vi "MCCETC_Status.vi"() -> (0 "n_ng":u8, 1 "values3":T1, 2 "values2":T2, 3 "values1":T3)   [LabVIEW 2019]
uses:
  MCCETC_Global.vi
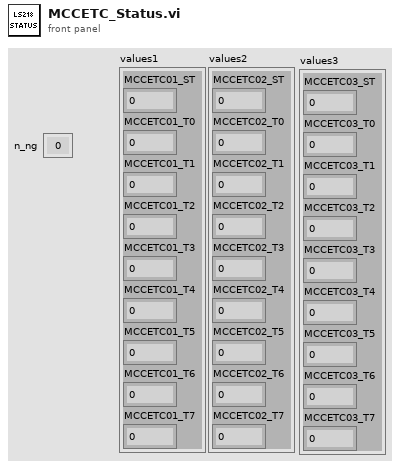
[diagram p1: front panel]
types:
  T1 = cluster{"MCCETC03_ST":u32, "MCCETC03_T0":dbl, "MCCETC03_T1":dbl, "MCCETC03_T2":dbl, "MCCETC03_T3":dbl, "MCCETC03_T4":dbl, "MCCETC03_T5":dbl, "MCCETC03_T6":dbl, "MCCETC03_T7":dbl}
  T2 = cluster{"MCCETC02_ST":u32, "MCCETC02_T0":dbl, "MCCETC02_T1":dbl, "MCCETC02_T2":dbl, "MCCETC02_T3":dbl, "MCCETC02_T4":dbl, "MCCETC02_T5":dbl, "MCCETC02_T6":dbl, "MCCETC02_T7":dbl}
  T3 = cluster{"MCCETC01_ST":u32, "MCCETC01_T0":dbl, "MCCETC01_T1":dbl, "MCCETC01_T2":dbl, "MCCETC01_T3":dbl, "MCCETC01_T4":dbl, "MCCETC01_T5":dbl, "MCCETC01_T6":dbl, "MCCETC01_T7":dbl}
  T4 = enum32{"Bad", "Idle", "Run top level", "Running"}
  T5 = cluster{"MKS670_1000_ST":u32, "MCCETC03_T0":dbl, "MCCETC03_T1":dbl, "MCCETC03_T2":dbl, "MCCETC03_T3":dbl, "MCCETC03_T4":dbl, "MCCETC03_T5":dbl, "MCCETC03_T6":dbl, "MCCETC03_T7":dbl}
  T6 = cluster{"MKS670_1000_ST":u32, "MCCETC02_T0":dbl, "MCCETC02_T1":dbl, "MCCETC02_T2":dbl, "MCCETC02_T3":dbl, "MCCETC02_T4":dbl, "MCCETC02_T5":dbl, "MCCETC02_T6":dbl, "MCCETC02_T7":dbl}
  T7 = cluster{"MKS670_1000_ST":u32, "MCCETC01_T0":dbl, "MCCETC01_T1":dbl, "MCCETC01_T2":dbl, "MCCETC01_T3":dbl, "MCCETC01_T4":dbl, "MCCETC01_T5":dbl, "MCCETC01_T6":dbl, "MCCETC01_T7":dbl}
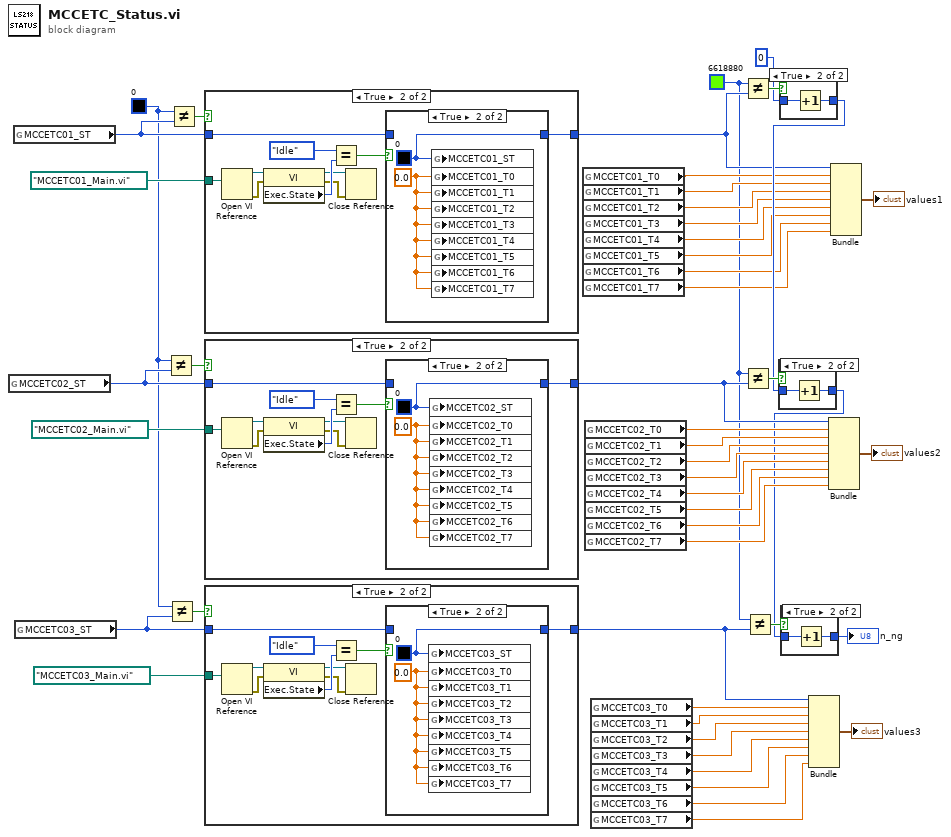
[diagram p0: block diagram]
diagram:
  w16 = u32 6618880 ("MKS670_1000_ST 2")
  w17 = u32 0 ("MKS670_1000_ST 2")
  n1 = global read "MCCETC_Global.vi" "MCCETC02_ST"() -> (w37:u32)
  n2 = global read "MCCETC_Global.vi" "MCCETC01_ST"() -> (w38:u32)
  n3 = global read "MCCETC_Global.vi" "MCCETC03_ST"() -> (w18:u32)
  n4 = Not Equal?(x=w17, y=w37) -> (x != y?=w46:bool)
  n5 = Not Equal?(x=w17, y=w18) -> (x != y?=w19:bool)
  n6 = Not Equal?(x=w17, y=w38) -> (x != y?=w48:bool)
  n7 = case shown="True" w48 {
    tunnel: w38 -> [w49 w51]
    tunnel: [w49 w50] -> w40
    tunnel: path "MCCETC01_Main.vi" ("vi path") -> [_ w52]
    frame False {
    }
    frame True {
      n8 = Open VI Reference(vi path=w52) -> (vi reference=w59:refnum<vi>, error out=w58:errorcluster)  [unwired: 5 in]
      n9 = property class="VI"(reference=w59, error in=w58) -> (reference out=w54:refnum<vi>, error out=w53:errorcluster, "Exec.State"=w56:T4)
      n10 = Equal?(x=T4."Idle" ("Execution:State"), y=w56) -> (x = y?=w57:bool)
      n11 = Close Reference(reference=w54, error in (no error)=w53) -> ()  [unwired: 1 out]
      n12 = case shown="True" w57 {
        tunnel: w51 -> [w60 _]
        tunnel: [w60 w62] -> w50
        frame False {
        }
        frame True {
          w61 = 0.0 ("MKS670_1000_P")
          w62 = u32 0 ("MKS670_1000_ST")
          n13 = global write "MCCETC_Global.vi" "MCCETC01_ST"(w62) -> ()
          n14 = global write "MCCETC_Global.vi" "MCCETC01_T0"(w61) -> ()
          n15 = global write "MCCETC_Global.vi" "MCCETC01_T1"(w61) -> ()
          n16 = global write "MCCETC_Global.vi" "MCCETC01_T2"(w61) -> ()
          n17 = global write "MCCETC_Global.vi" "MCCETC01_T3"(w61) -> ()
          n18 = global write "MCCETC_Global.vi" "MCCETC01_T4"(w61) -> ()
          n19 = global write "MCCETC_Global.vi" "MCCETC01_T5"(w61) -> ()
          n20 = global write "MCCETC_Global.vi" "MCCETC01_T6"(w61) -> ()
          n21 = global write "MCCETC_Global.vi" "MCCETC01_T7"(w61) -> ()
        }
      }
    }
  }
  n22 = case shown="True" w46 {
    tunnel: w37 -> [w63 w65]
    tunnel: [w63 w64] -> w39
    tunnel: path "MCCETC02_Main.vi" ("vi path") -> [_ w66]
    frame False {
    }
    frame True {
      n23 = Open VI Reference(vi path=w66) -> (vi reference=w73:refnum<vi>, error out=w72:errorcluster)  [unwired: 5 in]
      n24 = property class="VI"(reference=w73, error in=w72) -> (reference out=w68:refnum<vi>, error out=w67:errorcluster, "Exec.State"=w70:T4)
      n25 = Equal?(x=T4."Idle" ("Execution:State"), y=w70) -> (x = y?=w71:bool)
      n26 = Close Reference(reference=w68, error in (no error)=w67) -> ()  [unwired: 1 out]
      n27 = case shown="True" w71 {
        tunnel: w65 -> [w74 _]
        tunnel: [w74 w76] -> w64
        frame False {
        }
        frame True {
          w75 = 0.0 ("MKS670_1000_P")
          w76 = u32 0 ("MKS670_1000_ST")
          n28 = global write "MCCETC_Global.vi" "MCCETC02_ST"(w76) -> ()
          n29 = global write "MCCETC_Global.vi" "MCCETC02_T0"(w75) -> ()
          n30 = global write "MCCETC_Global.vi" "MCCETC02_T1"(w75) -> ()
          n31 = global write "MCCETC_Global.vi" "MCCETC02_T2"(w75) -> ()
          n32 = global write "MCCETC_Global.vi" "MCCETC02_T3"(w75) -> ()
          n33 = global write "MCCETC_Global.vi" "MCCETC02_T4"(w75) -> ()
          n34 = global write "MCCETC_Global.vi" "MCCETC02_T5"(w75) -> ()
          n35 = global write "MCCETC_Global.vi" "MCCETC02_T6"(w75) -> ()
          n36 = global write "MCCETC_Global.vi" "MCCETC02_T7"(w75) -> ()
        }
      }
    }
  }
  n37 = case shown="True" w19 {
    tunnel: w18 -> [w77 w79]
    tunnel: [w77 w78] -> w12
    tunnel: path "MCCETC03_Main.vi" ("vi path") -> [_ w80]
    frame False {
    }
    frame True {
      n38 = Open VI Reference(vi path=w80) -> (vi reference=w87:refnum<vi>, error out=w86:errorcluster)  [unwired: 5 in]
      n39 = property class="VI"(reference=w87, error in=w86) -> (reference out=w82:refnum<vi>, error out=w81:errorcluster, "Exec.State"=w84:T4)
      n40 = Equal?(x=T4."Idle" ("Execution:State"), y=w84) -> (x = y?=w85:bool)
      n41 = Close Reference(reference=w82, error in (no error)=w81) -> ()  [unwired: 1 out]
      n42 = case shown="True" w85 {
        tunnel: w79 -> [w88 _]
        tunnel: [w88 w90] -> w78
        frame False {
        }
        frame True {
          w89 = 0.0 ("MKS670_1000_P")
          w90 = u32 0 ("MKS670_1000_ST")
          n43 = global write "MCCETC_Global.vi" "MCCETC03_ST"(w90) -> ()
          n44 = global write "MCCETC_Global.vi" "MCCETC03_T0"(w89) -> ()
          n45 = global write "MCCETC_Global.vi" "MCCETC03_T1"(w89) -> ()
          n46 = global write "MCCETC_Global.vi" "MCCETC03_T2"(w89) -> ()
          n47 = global write "MCCETC_Global.vi" "MCCETC03_T3"(w89) -> ()
          n48 = global write "MCCETC_Global.vi" "MCCETC03_T4"(w89) -> ()
          n49 = global write "MCCETC_Global.vi" "MCCETC03_T5"(w89) -> ()
          n50 = global write "MCCETC_Global.vi" "MCCETC03_T6"(w89) -> ()
          n51 = global write "MCCETC_Global.vi" "MCCETC03_T7"(w89) -> ()
        }
      }
    }
  }
  n52 = global read "MCCETC_Global.vi" "MCCETC01_T0"() -> (w36:dbl)
  n53 = global read "MCCETC_Global.vi" "MCCETC01_T1"() -> (w35:dbl)
  n54 = global read "MCCETC_Global.vi" "MCCETC01_T2"() -> (w34:dbl)
  n55 = global read "MCCETC_Global.vi" "MCCETC01_T3"() -> (w33:dbl)
  n56 = global read "MCCETC_Global.vi" "MCCETC01_T4"() -> (w32:dbl)
  n57 = global read "MCCETC_Global.vi" "MCCETC01_T5"() -> (w31:dbl)
  n58 = global read "MCCETC_Global.vi" "MCCETC01_T6"() -> (w30:dbl)
  n59 = global read "MCCETC_Global.vi" "MCCETC01_T7"() -> (w29:dbl)
  n60 = global read "MCCETC_Global.vi" "MCCETC02_T0"() -> (w28:dbl)
  n61 = global read "MCCETC_Global.vi" "MCCETC02_T1"() -> (w27:dbl)
  n62 = global read "MCCETC_Global.vi" "MCCETC02_T2"() -> (w26:dbl)
  n63 = global read "MCCETC_Global.vi" "MCCETC02_T3"() -> (w25:dbl)
  n64 = global read "MCCETC_Global.vi" "MCCETC02_T4"() -> (w24:dbl)
  n65 = global read "MCCETC_Global.vi" "MCCETC02_T5"() -> (w23:dbl)
  n66 = global read "MCCETC_Global.vi" "MCCETC02_T6"() -> (w22:dbl)
  n67 = global read "MCCETC_Global.vi" "MCCETC02_T7"() -> (w21:dbl)
  n68 = global read "MCCETC_Global.vi" "MCCETC03_T0"() -> (w11:dbl)
  n69 = global read "MCCETC_Global.vi" "MCCETC03_T1"() -> (w4:dbl)
  n70 = global read "MCCETC_Global.vi" "MCCETC03_T2"() -> (w5:dbl)
  n71 = global read "MCCETC_Global.vi" "MCCETC03_T3"() -> (w6:dbl)
  n72 = global read "MCCETC_Global.vi" "MCCETC03_T4"() -> (w7:dbl)
  n73 = global read "MCCETC_Global.vi" "MCCETC03_T5"() -> (w8:dbl)
  n74 = global read "MCCETC_Global.vi" "MCCETC03_T6"() -> (w9:dbl)
  n75 = global read "MCCETC_Global.vi" "MCCETC03_T7"() -> (w10:dbl)
  n76 = Not Equal?(x=w16, y=w40) -> (x != y?=w44:bool)
  n77 = Not Equal?(x=w16, y=w39) -> (x != y?=w42:bool)
  n78 = Not Equal?(x=w16, y=w12) -> (x != y?=w15:bool)
  n79 = case shown="True" w44 {
    tunnel: u8 0 ("n_idle") -> [w91 w93]
    tunnel: [w91 w92] -> w41
    frame False {
    }
    frame True {
      n80 = Increment(x=w93) -> (x+1=w92:u8)
    }
  }
  n81 = case shown="True" w42 {
    tunnel: w41 -> [w94 w96]
    tunnel: [w94 w95] -> w14
    frame False {
    }
    frame True {
      n82 = Increment(x=w96) -> (x+1=w95:u8)
    }
  }
  n83 = case shown="True" w15 {
    tunnel: w14 -> [w97 w99]
    tunnel: [w97 w98] -> w13
    frame False {
    }
    frame True {
      n84 = Increment(x=w99) -> (x+1=w98:u8)
    }
  }
  "n_ng" <- w13
  n85 = Bundle("MKS670_1000_ST"=w12, "MCCETC03_T0"=w11, "MCCETC03_T1"=w4, "MCCETC03_T2"=w5, "MCCETC03_T3"=w6, "MCCETC03_T4"=w7, "MCCETC03_T5"=w8, "MCCETC03_T6"=w9, "MCCETC03_T7"=w10) -> (→"values3":T5)  [unwired: 1 in]
  n86 = Bundle("MKS670_1000_ST"=w39, "MCCETC02_T0"=w28, "MCCETC02_T1"=w27, "MCCETC02_T2"=w26, "MCCETC02_T3"=w25, "MCCETC02_T4"=w24, "MCCETC02_T5"=w23, "MCCETC02_T6"=w22, "MCCETC02_T7"=w21) -> (→"values2":T6)  [unwired: 1 in]
  n87 = Bundle("MKS670_1000_ST"=w40, "MCCETC01_T0"=w36, "MCCETC01_T1"=w35, "MCCETC01_T2"=w34, "MCCETC01_T3"=w33, "MCCETC01_T4"=w32, "MCCETC01_T5"=w31, "MCCETC01_T6"=w30, "MCCETC01_T7"=w29) -> (→"values1":T7)  [unwired: 1 in]
